vi "plot_init_panel.vi"(9 "Plot Tree":refnum<vi>, 10 "Window Title":refnum<vi>, 11 "Output Files Path":refnum<vi>) -> ()   [LabVIEW 2019]
uses:
  lib/libOutputReader/libOutputReader.lvlib
panel:
  out "Cluster":cluster{"1D array":string[][]}
  # "*******************************************************************\nBiogas Plant Control\n\nAuthor: Paul Zügel\nGCSC-Frankfurt am Main 2020\n\n*******************************************************************"
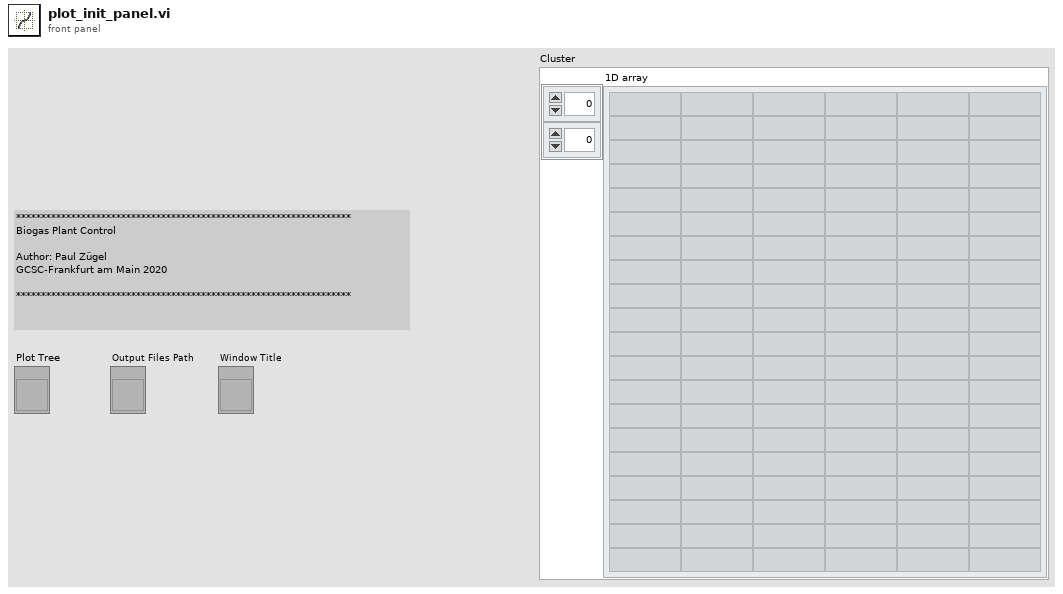
[diagram p1: front panel]
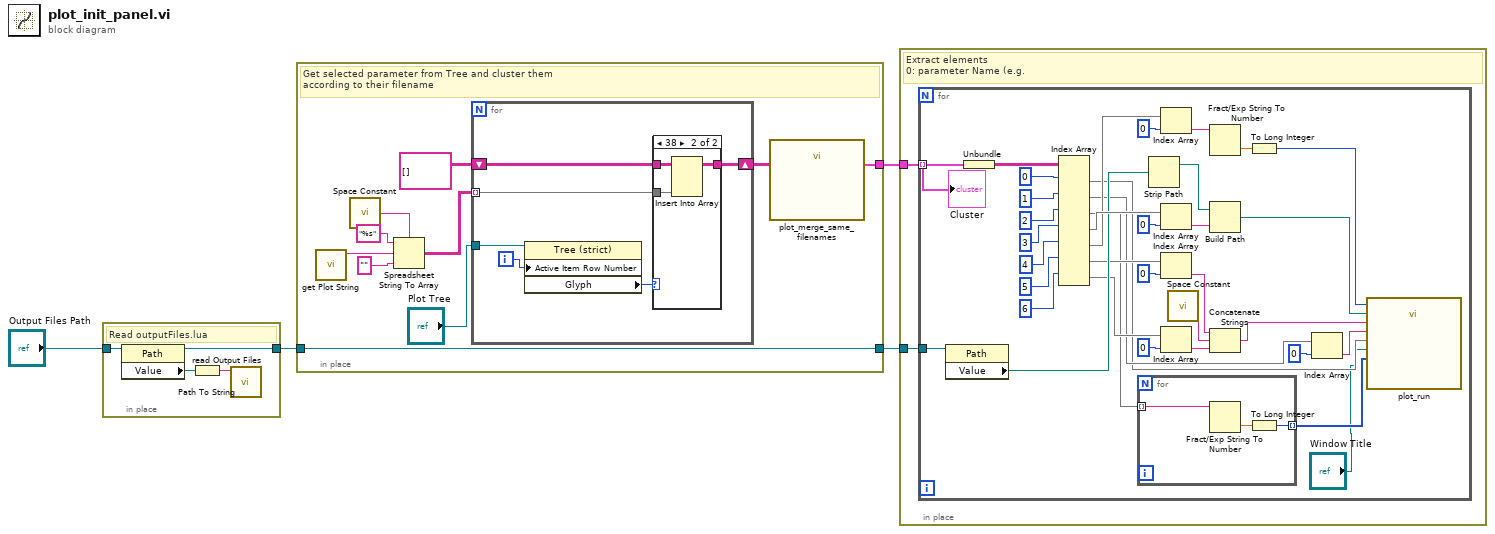
[diagram p0: block diagram]
diagram:
  n1 = in-place {
    in-place-border: "Output Files Path" -> [w8]
    in-place-border: [w5] -> w2
    # "Read outputFiles.lua"
    n2 = property class="Path"(reference=w8) -> (reference out=w5:refnum<vi>, "Value"=w7:path)  [unwired: 1 in, 1 out]
    n3 = Path To String(path=w7) -> (string=w6:string)
    n4 = call "read Output Files.vi"("path_to_outputFiles"=w6) -> ()  [unwired: 9 in, 2 out]
  }
  n5 = in-place {
    in-place-border: [w11] -> w3
    in-place-border: w2 -> [w9]
    in-place-border: [w9] -> w1
    # "Get selected parameter from Tree and cluster them\naccording to their filename"
    n6 = call "get Plot String.vi"() -> ("function return"=w15:string)  [unwired: 10 in, 1 out]
    n7 = call <vilib>:"Space Constant.vi"() -> ("String"=w16:string)
    n8 = Spreadsheet String To Array(delimiter (Tab)=w16, format string="%s", spreadsheet string=w15, array type (2D Dbl)="") -> (array=w14:string[][])
    n9 = for {
      tunnel: w14 -> [w19] mode=indexing
      shift-right: [w20] -> w12
      shift-left: string[][] [] -> [w21]
      tunnel: "Plot Tree" -> [w23]
      i -> [w24]
      n10 = property on="Property Node" class="Tree (strict)"(reference=w23, "Active Item Row Number"=w24) -> ("Glyph"=w22:i32)  [unwired: 1 in, 2 out]
      n11 = case shown="38" w22 {
        tunnel: w21 -> [w25 w28]
        tunnel: [w25 w27] -> w20
        tunnel: w19 -> [_ w26]
        frame 15, 37, Default {
        }
        frame 38 {
          n12 = Insert Into Array(array=w28, new element=w26) -> (w27:string[][])  [unwired: 2 in]
        }
      }
    }
    n13 = call "plot_merge_same_filenames.vi"("Input Array"=w12) -> ("Output Array"=w11:cluster{"1D array":string[][]}[])  [unwired: 10 in]
  }
  n14 = in-place {
    in-place-border: w1 -> [w30]
    in-place-border: w3 -> [w29]
    # "Extract elements\n0: parameter Name (e.g."
    n15 = for {
      tunnel: w29 -> [w59] mode=indexing
      tunnel: w30 -> [w54]
      n16 = property class="Path"(reference=w54) -> ("Value"=w55:path)  [unwired: 1 in, 2 out]
      n17 = Unbundle(w59) -> ("1D array"=w58:string[][])
      n18 = Index Array(array=w58, index (row) #1=0 ("index (row)"), index (row) #2=1 ("index (row)"), index (row) #3=2 ("index (row)"), index (row) #4=3 ("index (row)"), index (row) #5=4 ("index (row)"), index (row) #6=5 ("index (row)"), index (row) #7=6 ("index (row)")) -> (element #1=w32:string[], element #2=w35:string[], element #3=w37:string[], element #4=w57:string[], element #5=w48:string[], element #6=w45:string[], element #7=w44:string[])  [unwired: 7 in]
      n19 = for {
        tunnel: w37 -> [w68] mode=indexing
        tunnel: [w67] -> w36 mode=indexing
        n20 = Fract/Exp String To Number(string=w68) -> (number=w69:dbl)  [unwired: 3 in, 1 out]
        n21 = To Long Integer(number=w69) -> (32bit integer=w67:i32)
      }
      n22 = Strip Path(path=w55) -> (stripped path=w53:path)  [unwired: 1 out]
      n23 = Index Array(array=w48, index=0) -> (element=w46:string)
      n24 = Index Array(array=w57, index=0) -> (element=w52:string)
      n25 = Index Array(array=w45, index=0) -> (element=w41:string)
      n26 = Index Array(array=w44, index=0) -> (element=w40:string)
      n27 = call <vilib>:"Space Constant.vi"() -> ("String"=w39:string)
      n28 = Fract/Exp String To Number(string=w46) -> (number=w50:dbl)  [unwired: 3 in, 1 out]
      n29 = Build Path(base path=w53, name or relative path=w52) -> (appended path=w51:path)
      n30 = Concatenate Strings(w41, w39, w40) -> (w38:string)
      n31 = To Long Integer(number=w50) -> (32bit integer=w49:i32)
      n32 = Index Array(array=w35, index=0) -> (element=w33:string)
      n33 = call "plot_run.vi"("xValues"=w49, "yValues"=w36, "File Path"=w51, "xName"=w38, "yName"=w33, "Window Title"="Window Title", "yNames"=w32) -> ()  [unwired: 4 in]
      "Cluster" <- w59
    }
  }
